vi "Spatial Dual Decode Packet 50 (SubVI).vi"(7 "Unix Timestamp":u64, 8 "SGL Precision":i16=6, 10 "Packet 50 Bytes In":u8[](array[numeric])) -> (0 "Channel Data Type":string[](array[string])=["Float", "Float", "Float"], 1 "Channel Units":string[](array[string])=["m/s/s", "m/s/s", "m/s/s"], 2 "Data":string[](array[string]), 3 "Channel Names":string[](array[string])=["Acc X", "Acc Y", "Acc Z"], 4 "Packet 50 Decoded Data Cluster":T1)   [LabVIEW 2019, in "SpatialDual_Parsers.lvlib"]
uses:
  SpatialDual_Parsers.lvlib
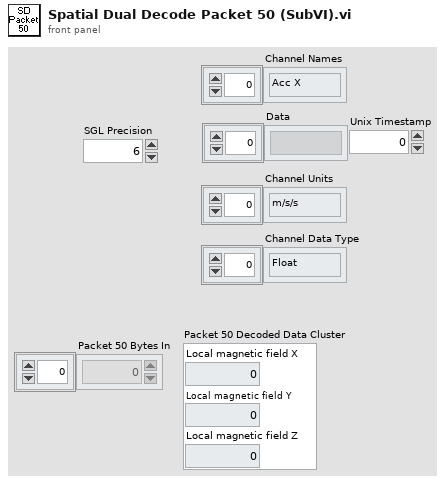
[diagram p1: front panel]
types:
  T1 = cluster{"Local magnetic field X":sgl, "Local magnetic field Y":sgl, "Local magnetic field Z":sgl}
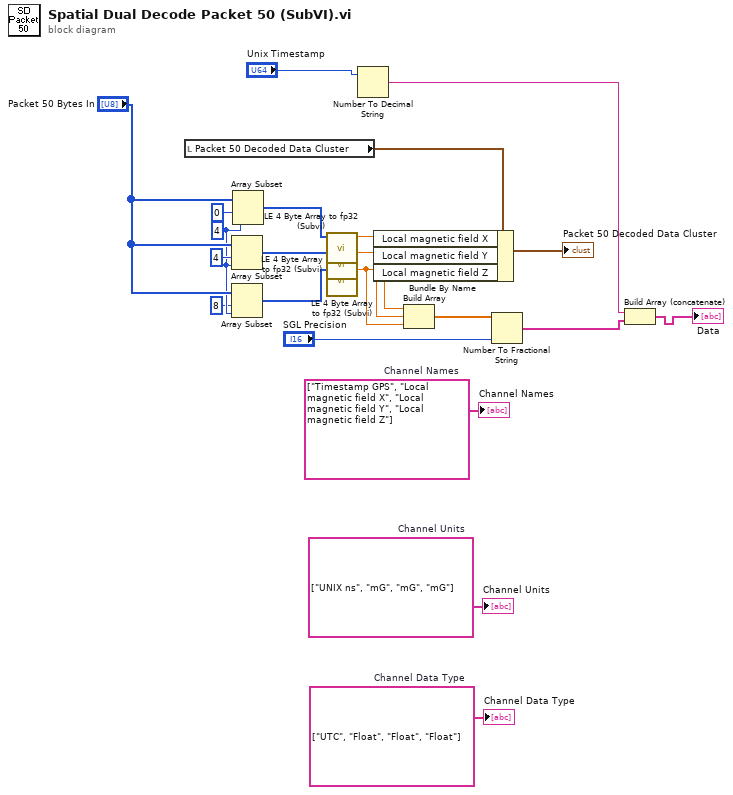
[diagram p0: block diagram]
diagram:
  w5 = string[] ["UTC", "Float", "Float", "Float"]  # Channel Data Type
  w6 = string[] ["UNIX ns", "mG", "mG", "mG"]  # Channel Units
  w7 = string[] ["Timestamp GPS", "Local magnetic field X", "Local magnetic field Y", "Local magnetic field Z"]  # Channel Names
  w17 = 4 ("length")
  n1 = local read "Packet 50 Decoded Data Cluster"() -> (w22:T1)
  n2 = Array Subset(array="Packet 50 Bytes In", index=4, length=w17) -> (w14:u8[])
  n3 = Array Subset(array="Packet 50 Bytes In", index=8, length=w17) -> (w15:u8[])
  n4 = Array Subset(array="Packet 50 Bytes In", index=0, length=w17) -> (w13:u8[])
  n5 = call "LE 4 Byte Array to fp32 (Subvi).vi"("4 Bytes in"=w13) -> ("fp32 Out"=w12:sgl)  [unwired: 8 in]
  n6 = call "LE 4 Byte Array to fp32 (Subvi).vi"("4 Bytes in"=w14) -> ("fp32 Out"=w11:sgl)  [unwired: 8 in]
  n7 = call "LE 4 Byte Array to fp32 (Subvi).vi"("4 Bytes in"=w15) -> ("fp32 Out"=w10:sgl)  [unwired: 8 in]
  n8 = Number To Decimal String(number="Unix Timestamp") -> (decimal integer string=w1:string)  [unwired: 1 in]
  n9 = Bundle By Name(cluster=w22, "Local magnetic field X"=w12, "Local magnetic field Y"=w11, "Local magnetic field Z"=w10) -> (→"Packet 50 Decoded Data Cluster":T1)
  n10 = Build Array(w12, w11, w10) -> (w9:sgl[])
  n11 = Number To Fractional String(number=w9, precision (6)="SGL Precision") -> (F-format string=w4:string[])  [unwired: 2 in]
  n12 = Build Array (concatenate)(w1, w4) -> (→"Data":string[])
  "Channel Names" <- w7
  "Channel Units" <- w6
  "Channel Data Type" <- w5
